vi "Update_DestDir_For_Main_Dest_Change.vi"(8 "error in (no error)":errorcluster, 10 "strip file name? (T)":bool=TRUE, 11 "Build in":refnum<class "AB_Build.lvclass">) -> (0 "error out":errorcluster, 3 "Build out":refnum<class "AB_Build.lvclass">)   [LabVIEW 2020, in "AB_Deployment.lvlib"]
uses:
  <vilib>/AppBuilder/AB_Classes/Deployment/AB_Deployment.lvlib
  <vilib>/AppBuilder/AB_Classes/Build/AB_Build.lvclass
  <vilib>/AppBuilder/AB_Classes/Destination/AB_Destination.lvclass
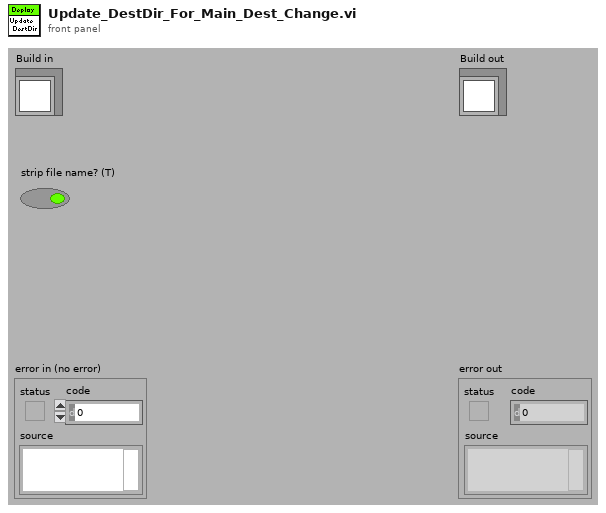
[diagram p1: front panel]
types:
  T1 = typedef "AB_Build.ctl" = cluster{"buildSpecName":string, "buildSpecDescription":string, "destinations":refnum<class "AB_Destination.lvclass">[], "exclusionOption":T2, "defaultLanguage":string, "supportedLanguages":string[], "excludedDirectories":path[], "buildContext":refnum<vi>, "buildObject":T3, "preview":bool, "programatic":bool, "progressBarEvents":T4, "userLog_Path":path, "preActionID":string, "preAction_Path":path, "postActionID":string, "postAction_Path":path, "eng_checkForBrokenVIs?":bool, "eng_verboseLinkerErrors?":bool, "localDest_Path":path, "targetDest_Path":path, "removeVIObject":u16, "cache":refnum<class "PreviewCache.lvclass">, "use cache":bool, "previewCache_ID":string, "buildCache_ID":string, "eng_TempLocalDest_Path":path, "eng_collectDependencies?":bool, "versionInfo":cluster{"buildVersion":cluster{"major":u16, "minor":u16, "patch":u16, "build":u16}, "autoIncrement":bool}, "eng_enableVIChecksums":bool}
  T2 = typedef "AB_Exclusion_Option.ctl" = cluster{"typedefs":bool, "polymorphicVIs":bool, "unusedLibraryItems":bool, "modifyLibraryFile":bool, "edit-timeDependencies":bool, "inlineVIs":bool, "dependent PPLs":bool, "dependent DLLs":bool}
  T3 = typedef "ItemRef.ctl" = u64
  T4 = typedef "provcom_ProgressBar_Events.ctl" = cluster{"newJob":refnum<user-event>, "newItem":refnum<user-event>, "errorMsg":T5, "cancel":refnum<user-event>}
  T5 = typedef "mxLvBuildError.ctl" = refnum<user-event>
  T6 = typedef "AB_Destination.ctl" = cluster{"destName":string, "path":path, "libraryName":string, "preserveHierarchy":bool, "eng_inBuild":bool, "eng_libraryReference":refnum<vi>, "eng_restictAddToNewLibrary":bool}
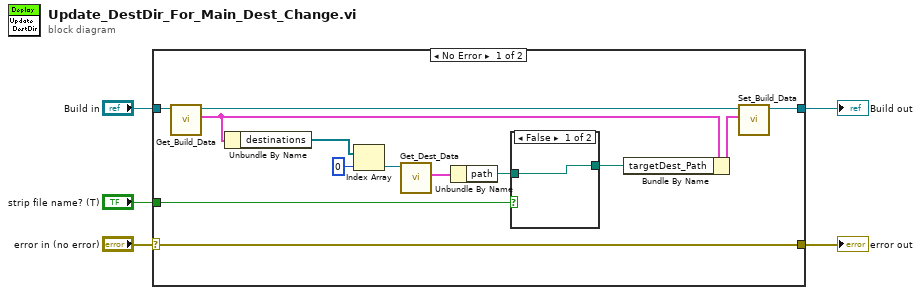
[diagram p0: block diagram]
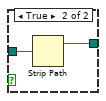
[diagram p2: hidden frame]
diagram:
  n1 = case shown="No Error" "error in (no error)" {
    selector: "error in (no error)" -> [w18 w23]
    tunnel: [w18 w23] -> w3
    tunnel: [w12 w22] -> w4
    tunnel: "Build in" -> [w13 w22]
    tunnel: "strip file name? (T)" -> [w6 _]
    frame No Error {
      n2 = call <vilib>:"Get_Build_Data.vi"("Class in"=w13) -> ("data"=w11:T1, "Class out"=w10:refnum<class "AB_Build.lvclass">)  [unwired: 8 in, 1 out]
      n3 = Unbundle By Name(w11) -> ("destinations"=w17:refnum<class "AB_Destination.lvclass">[])
      n4 = Index Array(array=w17, index=0) -> (element=w15:refnum<class "AB_Destination.lvclass">)
      n5 = call <vilib>:"Get_Dest_Data.vi"("Class in"=w15) -> ("destName"=w14:T6)  [unwired: 8 in, 2 out]
      n6 = Unbundle By Name(w14) -> ("path"=w8:path)
      n7 = case shown="False" w6 {
        tunnel: w8 -> [w19 w21]
        tunnel: [w19 w20] -> w7
        frame False {
        }
        frame True {
          n8 = Strip Path(path=w21) -> (stripped path=w20:path)  [unwired: 1 out]
        }
      }
      n9 = Bundle By Name(cluster=w11, "targetDest_Path"=w7) -> (w9:T1)
      n10 = call <vilib>:"Set_Build_Data.vi"("data"=w9, "Class in"=w10) -> ("Class out"=w12:refnum<class "AB_Build.lvclass">)  [unwired: 8 in, 1 out]
    }
    frame Error {
    }
  }
  "error out" <- w3
  "Build out" <- w4
